vi "Normalised_Autocorrelation.vi"(1 "Autocorrelation length":i32, 2 "Array":dbl[](array[numeric]) format="%.2f") -> (0 "Normalised Auto corr":dbl[](array[numeric]) format="%.2f")   [LabVIEW 2020]
uses:
  <vilib>/Analysis/baseanly.llb/Mean (DBL).vi
  <vilib>/Analysis/NI_AALBase.lvlib
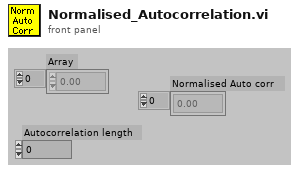
[diagram p1: front panel]
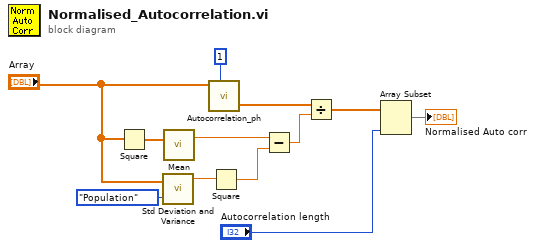
[diagram p0: block diagram]
diagram:
  n1 = Square(x="Array") -> (x^2=w10:dbl[])
  n2 = call <vilib>:"Std Deviation and Variance.vi"("X"="Array", "Weighting (Sample)"=enum16{"Sample", "Population"}."Population") -> ("mean"=w9:dbl)  [unwired: 2 out]
  n3 = call-poly <vilib>:"Mean.vi"("X"=w10) -> ("mean"=w7:dbl)  [unwired: 1 out]
  n4 = call "Autocorrelation_ph.vi"("X"="Array", "Block No"=1) -> ("Autocorrelation of X"=w4:dbl[])  [unwired: 4 in]
  n5 = Square(x=w9) -> (x^2=w8:dbl)
  n6 = Subtract(x=w7, y=w8) -> (x-y=w3:dbl)
  n7 = Divide(x=w4, y=w3) -> (x/y=w2:dbl[])
  n8 = Array Subset(array=w2, length="Autocorrelation length") -> (→"Normalised Auto corr":dbl[])  [unwired: 1 in]
